vi "纳清电导率_所有参数读取.vi"(8 "error in (no error)":errorcluster caption="错误输入（无错误）", 11 "MB session in":refnum<class "MB_Master.lvclass">) -> (0 "error out":errorcluster caption="错误输出", 2 "输出值":T1 {"波特率" items=["4800", "9600", "19200", "38400", "57600", "115200"]}, 3 "MB session out":refnum<class "MB_Master.lvclass">)   [LabVIEW 2016, in "斯坦道多参数.lvlib"]
uses:
  <vilib>/Plasmionique/MB Master/MB_Master/MB_Master.lvclass
  <vilib>/Plasmionique/MB Master/MB Master.lvlib
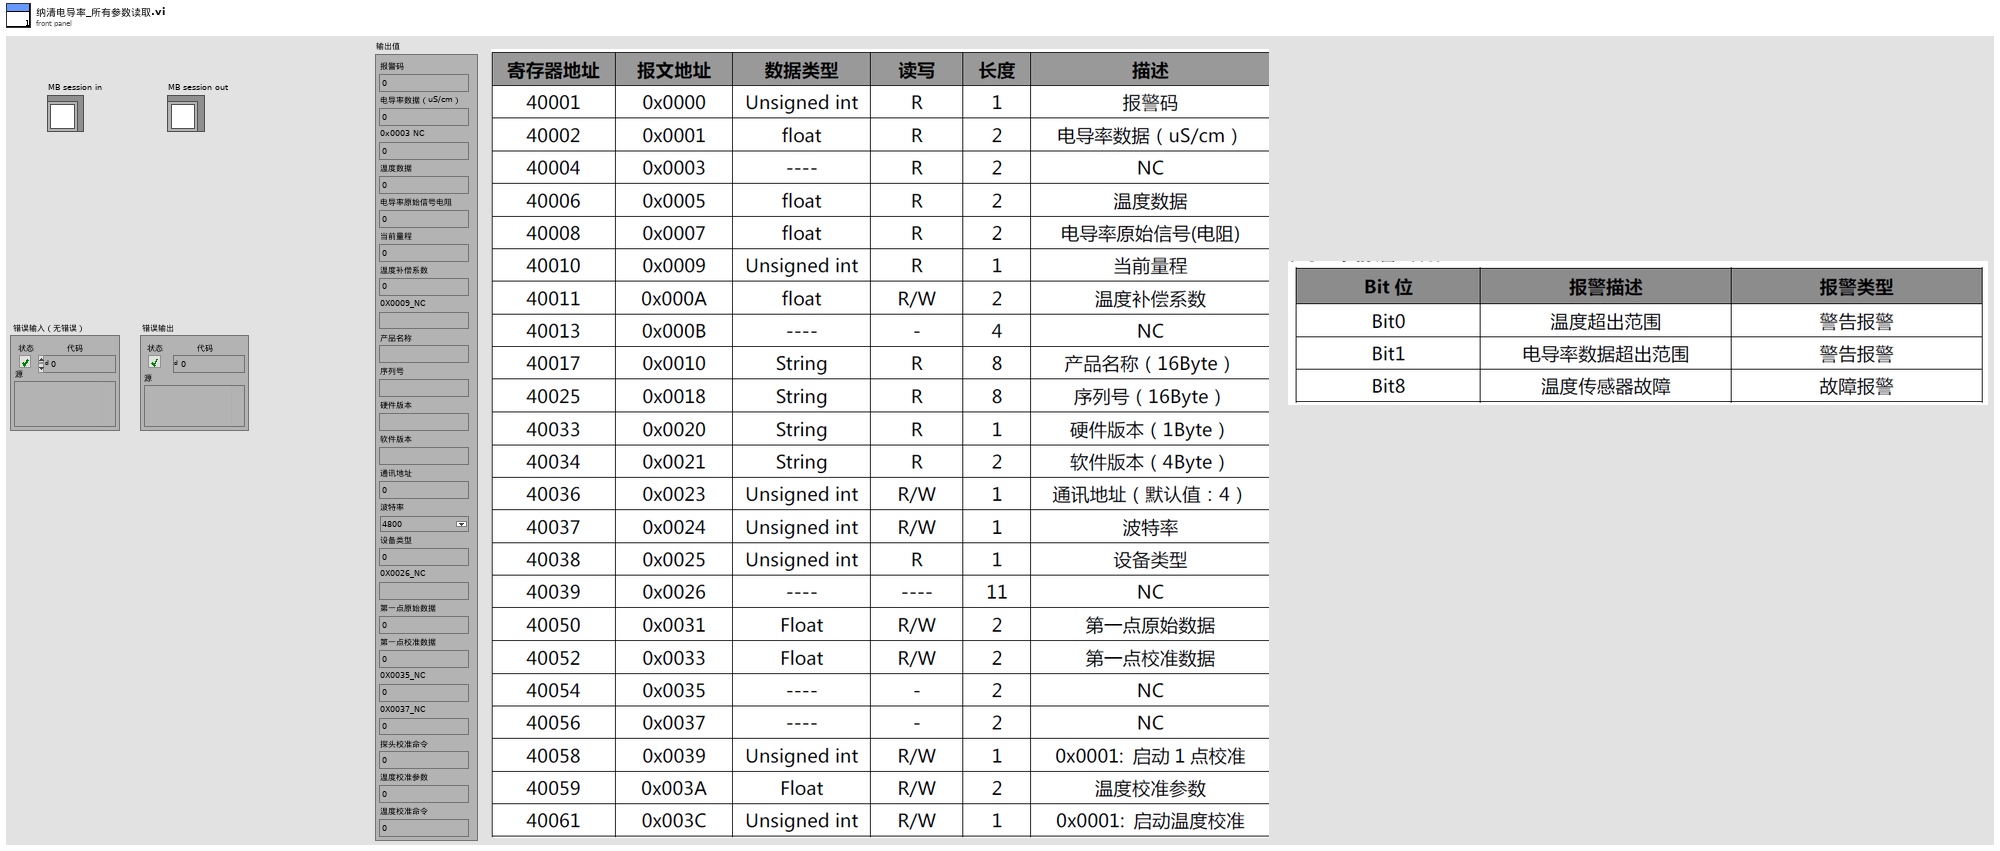
[diagram p1: front panel]
types:
  T1 = cluster{"报警码":u16, "电导率数据（uS/cm）":sgl, "0x0003 NC":sgl, "温度数据":sgl, "电导率原始信号电阻":sgl, "当前量程":u16, "温度补偿系数":sgl, "0X0009_NC":string, "产品名称":string, "序列号":string, "硬件版本":string, "软件版本":string, "通讯地址":u16, "波特率":u16, "设备类型":u16, "0X0026_NC":string, "第一点原始数据":sgl, "第一点校准数据":sgl, "0X0035_NC":sgl, "0X0037_NC":sgl, "探头校准命令":u16, "温度校准参数":sgl, "温度校准命令":u16}
  T2 = cluster{u16, "mode":dbl, "数值":sgl, "数值":sgl, "数值":sgl, u16, "数值":sgl, "类型":string, "类型":string, "类型":string, "类型":string, "类型":string, u16, u16, u16, "类型":string, "数值":sgl, "数值":sgl, "数值":sgl, "数值":sgl, u16, "数值":sgl, u16}
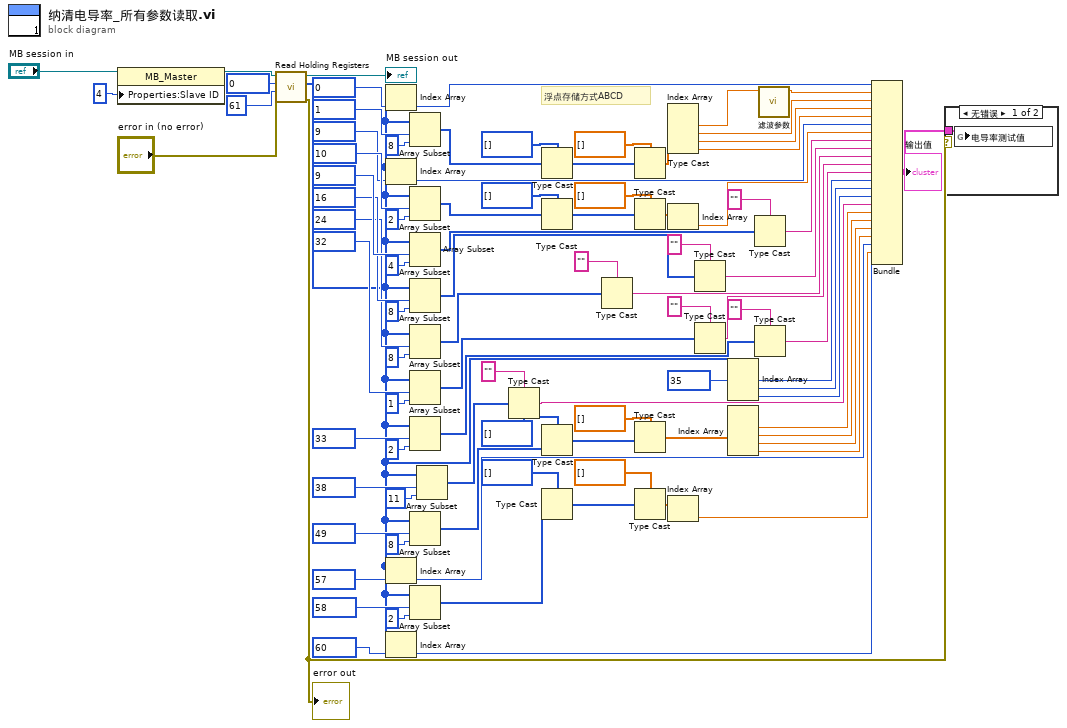
[diagram p0: block diagram]
diagram:
  # "浮点存储方式ABCD"
  n1 = property class="MB_Master"(reference="MB session in", "Properties:Slave ID"=u8 4 ("Slave ID")) -> (reference out=w81:refnum<class "MB_Master.lvclass">)  [unwired: 1 in, 1 out]
  n2 = call <vilib>:"Read Holding Registers.vi"("error in (no error)"="error in (no error)", "quantity"=u16 61, "starting address"=u16 0, "MB session in"=w81) -> ("error out"=w23:errorcluster, "Registers"=w4:u16[], "MB session out"=→"MB session out":refnum<class "MB_Master.lvclass">)  [unwired: 5 in]
  "error out" <- w23
  n3 = Index Array(array=w4, index=u16 0 ("starting address")) -> (element=w89:u16)
  n4 = Index Array(array=w4, index=u16 9 ("starting address")) -> (element=w3:u16)
  n5 = Index Array(array=w4, index=u16 57 ("starting address")) -> (element=w27:u16)
  n6 = Index Array(array=w4, index=u16 60 ("starting address")) -> (element=w24:u16)
  n7 = Array Subset(array=w4, index=u16 1 ("starting address"), length=8 ("长度")) -> (w85:u16[])
  n8 = Array Subset(array=w4, index=u16 10 ("starting address"), length=2 ("长度")) -> (w7:u16[])
  n9 = Array Subset(array=w4, index=u16 9 ("starting address"), length=4 ("长度")) -> (w75:u16[])
  n10 = Array Subset(array=w4, index=u16 16 ("starting address"), length=8 ("长度")) -> (w71:u16[])
  n11 = Array Subset(array=w4, index=u16 24 ("starting address"), length=8 ("长度")) -> (w65:u16[])
  n12 = Array Subset(array=w4, index=u16 32 ("starting address"), length=1 ("长度")) -> (w61:u16[])
  n13 = Array Subset(array=w4, index=u16 33 ("starting address"), length=2 ("长度")) -> (w55:u16[])
  n14 = Array Subset(array=w4, index=u16 49 ("starting address"), length=8 ("长度")) -> (w42:u16[])
  n15 = Array Subset(array=w4, index=u16 58 ("starting address"), length=2 ("长度")) -> (w30:u16[])
  n16 = Array Subset(array=w4, index=u16 38 ("starting address"), length=11 ("长度")) -> (w45:u16[])
  n17 = Type Cast(type="" ("类型"), x=w45) -> (*(type *) &x=w44:string)
  n18 = Type Cast(type=u32[] [] ("数组 2"), x=w85) -> (*(type *) &x=w22:u32[])
  n19 = Type Cast(type=u32[] [] ("数组 2"), x=w7) -> (*(type *) &x=w11:u32[])
  n20 = Type Cast(type=u32[] [] ("数组 2"), x=w42) -> (*(type *) &x=w40:u32[])
  n21 = Type Cast(type=u32[] [] ("数组 2"), x=w30) -> (*(type *) &x=w32:u32[])
  n22 = Type Cast(type="" ("类型"), x=w65) -> (*(type *) &x=w63:string)
  n23 = Type Cast(type=sgl[] [] ("数组 2"), x=w22) -> (*(type *) &x=w84:sgl[])
  n24 = Type Cast(type=sgl[] [] ("数组 2"), x=w11) -> (*(type *) &x=w10:sgl[])
  n25 = Type Cast(type=sgl[] [] ("数组 2"), x=w40) -> (*(type *) &x=w37:sgl[])
  n26 = Type Cast(type=sgl[] [] ("数组 2"), x=w32) -> (*(type *) &x=w35:sgl[])
  n27 = Index Array(array=w84) -> (element #1=w2:sgl, element #2=w79:sgl, element #3=w19:sgl, element #4=w18:sgl)  [unwired: 4 in]
  n28 = Index Array(array=w10) -> (element=w6:sgl)  [unwired: 1 in]
  n29 = Index Array(array=w35) -> (element=w26:sgl)  [unwired: 1 in]
  n30 = Type Cast(type="" ("类型"), x=w71) -> (*(type *) &x=w68:string)
  n31 = Type Cast(type="" ("类型"), x=w61) -> (*(type *) &x=w58:string)
  n32 = Index Array(array=w4, index #1=u16 35 ("starting address")) -> (element #1=w51:u16, element #2=w50:u16, element #3=w49:u16)  [unwired: 2 in]
  n33 = Index Array(array=w37) -> (element #1=w36:sgl, element #2=w17:sgl, element #3=w16:sgl, element #4=w15:sgl)  [unwired: 4 in]
  n34 = Type Cast(type="" ("类型"), x=w75) -> (*(type *) &x=w73:string)
  n35 = Type Cast(type="" ("类型"), x=w55) -> (*(type *) &x=w53:string)
  n36 = call "滤波参数.vi"("x"=w2) -> ("mode"=w1:dbl)  [unwired: 10 in]
  n37 = Bundle(w89, "mode"=w1, "数值"=w79, "数值"=w19, "数值"=w18, w3, "数值"=w6, "类型"=w73, "类型"=w68, "类型"=w63, "类型"=w58, "类型"=w53, w51, w50, w49, "类型"=w44, "数值"=w36, "数值"=w17, "数值"=w16, "数值"=w15, w27, "数值"=w26, w24) -> (w14:T2)  [unwired: 1 in]
  "输出值" <- w14
  n38 = case shown="无错误" w23 {
    tunnel: w14 -> [w92 _]
    frame No Error {
      n39 = global write "纳清过程全局变量.vi" "电导率测试值"(w92) -> ()
    }
    frame Error {
    }
  }
